vi "enter-registration2.vi"(0 "Array input":string[](array[string])) -> (1 "Array output":string[](array[string]), 2 "Numeric":dbl)   [LabVIEW 2023]
panel:
  in  "OK":bool caption="ZATWIERDZ"
  in  "registration":string caption="Wprowadz rejestracje"
  # "Wpisz numery rejestracyjne twojego samochodu, a nastepnie nacisni ZATWIERDZ"
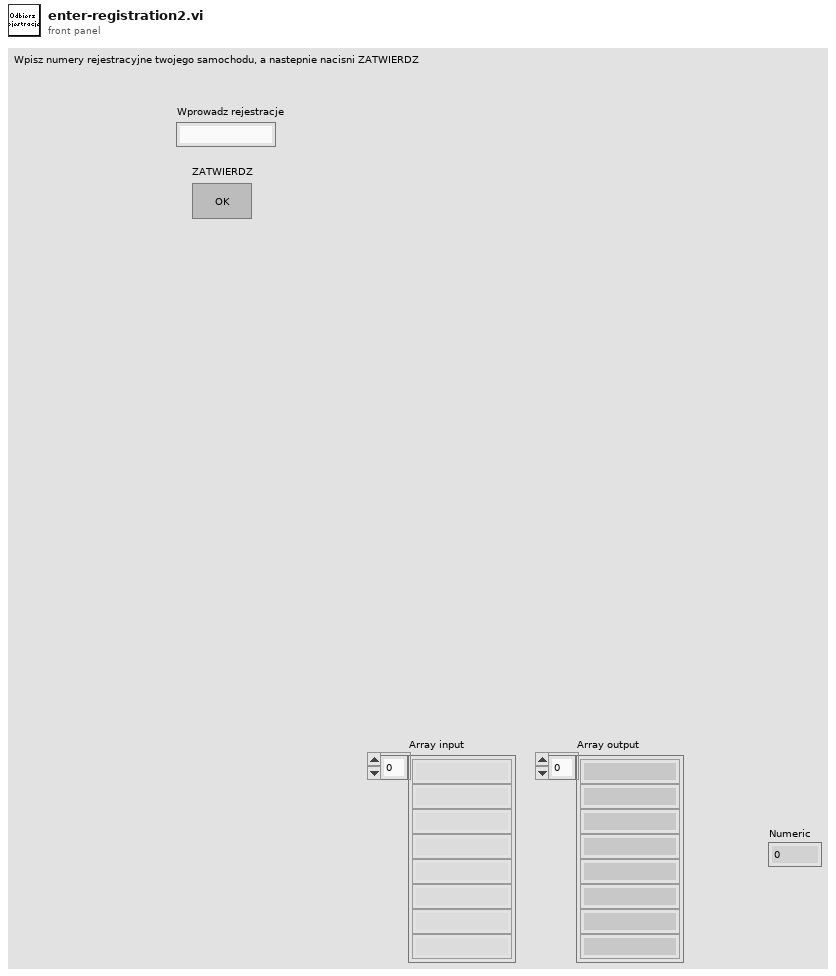
[diagram p1: front panel]
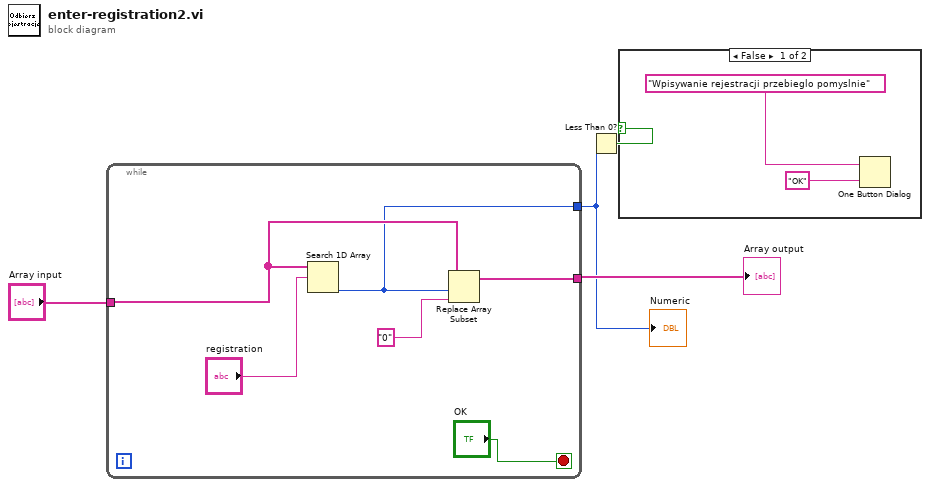
[diagram p0: block diagram]
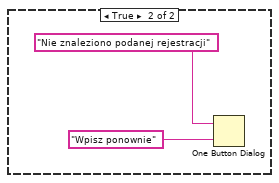
[diagram p2: hidden frame]
diagram:
  n1 = while {
    tunnel: "Array input" -> [w6]
    tunnel: [w7] -> w3
    tunnel: [w5] -> w1
    stop <- "OK" stop-if-true
    n2 = Search 1D Array(1D array=w6, element="registration") -> (index of element=w5:i32)  [unwired: 1 in]
    n3 = Replace Array Subset(array=w6, new element="0" ("new element/subarray"), index=w5) -> (w7:string[])
  }
  "Array output" <- w3
  "Numeric" <- w1
  n4 = Less Than 0?(x=w1) -> (x < 0?=w2:bool)
  n5 = case shown="False" w2 {
    frame False {
      n6 = One Button Dialog(message="Wpisywanie rejestracji przebieglo pomyslnie", button name ("OK")="OK") -> ()  [unwired: 1 out]
    }
    frame True {
      n7 = One Button Dialog(message="Nie znaleziono podanej rejestracji", button name ("OK")="Wpisz ponownie") -> ()  [unwired: 1 out]
    }
  }
